vi "Get Match ID.vi"(0 "Refnum in":refnum<k35>, 2 "mode":string, 3 "error in (no error)":errorcluster) -> (6 "Refnum out":refnum<k35>, 7 "return value":string, 8 "is_ok":errorcluster, 10 "error out":errorcluster)   [LabVIEW 2025]
panel:
  out "s? t:f":errorcluster
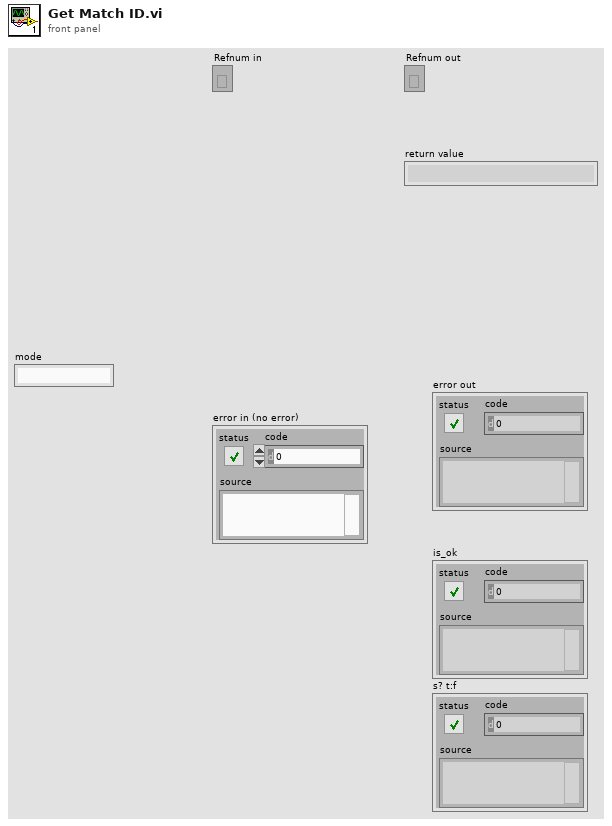
[diagram p1: front panel]
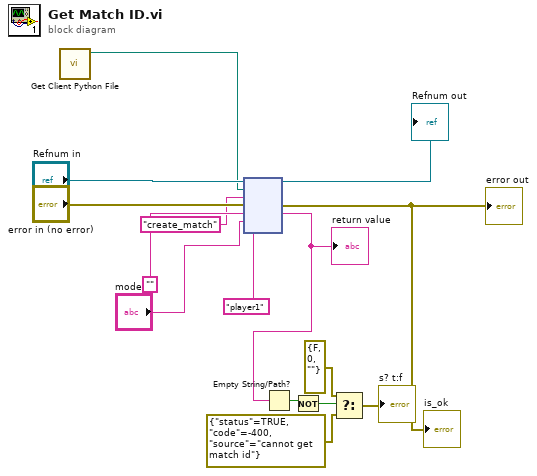
[diagram p0: block diagram]
diagram:
  n1 = call "Get Client Python File.vi"() -> ("appended path"=w4:path)  [unwired: 11 in]
  n2 = node("Refnum in", w4, "create_match" ("function name"), "error in (no error)", "", "mode", "player1") -> (→"Refnum out":refnum<k35>, →"is_ok" →"error out":errorcluster, w13:string)  [unwired: 2 in, 2 out]
  "return value" <- w13
  n3 = Empty String/Path?(string/path=w13) -> (empty?=w14:bool)
  n4 = Not(x=w14) -> (.not. x?=w15:bool)
  n5 = Select(t=errorcluster {"status"=FALSE, "code"=0, "source"=""} ("error constant"), s=w15, f=errorcluster {"status"=TRUE, "code"=-400, "source"="cannot get match id"} ("error constant")) -> (s? t:f=→"s? t:f":errorcluster)
